vi "Perform Work.vi"(4 "Controller name":string, 6 "Last request":bool, 7 "Update period":dbl, 8 "error in (no error)":errorcluster, 9 "Initialize":bool, 11 "Measure Controller in":refnum<class "Pulse Controller.lvclass">) -> (0 "error out":errorcluster, 3 "Measure Controller out":refnum<class "Pulse Controller.lvclass">)   [LabVIEW 2021, in "Pulse Controller.lvclass"]
uses:
  Pulse Controller.lvclass
  C:/GitHub/LabActor/Template Module/Template Module.lvclass
  C:/GitHub/LabActor/Controllers/Process Controller/Process Controller.lvclass
  Template Module/Template Module.lvclass/Template Module.ctl
  Process Controller/Process Controller.lvclass/Process Controller.ctl
  Pulse Recorders/Interfaces/Pulse Recorder Messages/Arm Msg/Arm Msg.lvclass/Arm Msg.ctl
  <vilib>/ActorFramework/Message Enqueuer/Message Enqueuer.lvclass/Message Enqueuer.ctl
  Template Module/Read tdms stream.vi
  Process Controller/Read Active measurements enqueuers.vi
  <vilib>/ActorFramework/Message Enqueuer/Enqueue.vi
  Pulse Recorders/Interfaces/Pulse Recorder Messages/Arm Msg/Arm Msg.lvclass
  C:/Program Files/National Instruments/LabVIEW 2021/vi.lib/ActorFramework/Message/Message.lvclass
  <vilib>/ActorFramework/Message Priority Queue/Priority Enqueue.vi
  Process Controller/Process Controller.lvclass
  <vilib>/ActorFramework/Message Enqueuer/Message Enqueuer.lvclass
panel:
  out "NaN/Path/Refnum? 2":bool
  out "NaN/Path/Refnum?":bool
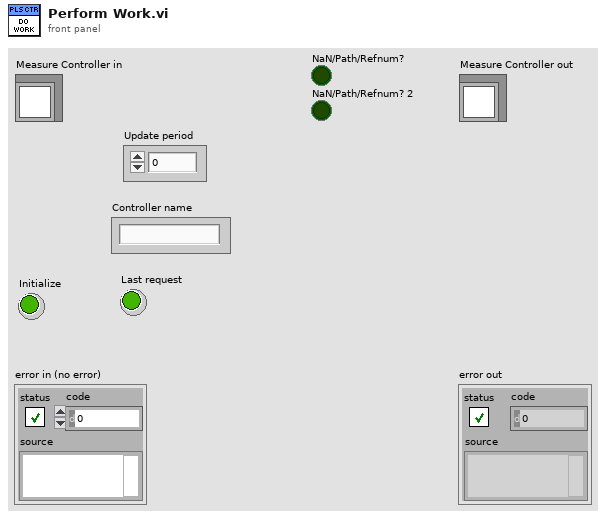
[diagram p1: front panel]
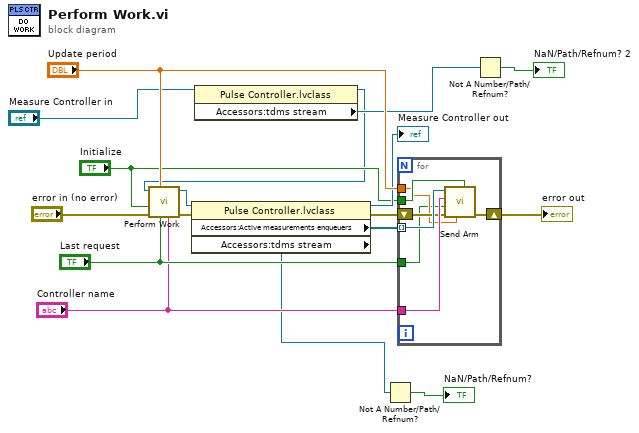
[diagram p0: block diagram]
diagram:
  n1 = property class="Pulse Controller.lvclass"(reference="Measure Controller in") -> (reference out=w1:refnum<class "Pulse Controller.lvclass">, "Accessors:tdms stream"=w2:refnum<k34>)  [unwired: 1 in, 1 out]
  n2 = call-parent "Perform Work.vi"("Controller name"="Controller name", "Last request"="Last request", "Update period"="Update period", "error in (no error)"="error in (no error)", "Initialize"="Initialize", "Measure Controller in"=w1) -> ("error out"=w13:errorcluster, "Measure Controller out"=w14:refnum<class "Pulse Controller.lvclass">)  [unwired: 4 in]
  n3 = property class="Pulse Controller.lvclass"(reference=w14, error in=w13) -> (reference out=→"Measure Controller out":refnum<class "Pulse Controller.lvclass">, error out=w16:errorcluster, "Accessors:Active measurements enqueuers"=w15:refnum<class "Message Enqueuer.lvclass">[], "Accessors:tdms stream"=w5:refnum<k34>)
  n4 = Not A Number/Path/Refnum?(number/path/refnum=w5) -> (NaN/Path/Refnum?=→"NaN/Path/Refnum?":bool)
  n5 = for {
    tunnel: w15 -> [w23] mode=indexing
    tunnel: "Controller name" -> [w24]
    shift-right: [w21] -> w7
    shift-left: w16 -> [w22]
    tunnel: "Update period" -> [w19]
    tunnel: "Last request" -> [w18]
    tunnel: "Initialize" -> [w20]
    n6 = call "Send Arm.vi"("Init work"=w20, "Update period"=w19, "error in (no error)"=w22, "Last request"=w18, "Requester"=w24, "Message Enqueuer"=w23) -> ("error out"=w21:errorcluster)  [unwired: 4 in, 1 out]
  }
  "error out" <- w7
  n7 = Not A Number/Path/Refnum?(number/path/refnum=w2) -> (NaN/Path/Refnum?=→"NaN/Path/Refnum? 2":bool)
